vi "HHSetInpChan.vi"(0 "Channel":i32=1 min=1 max=8 step=1, 1 "CFD Level":i32=50 min=-1300 max=400 step=10, 2 "CFD ZeroX":i32=10 min=-1300 max=400 step=10, 3 "Offset":i32=10 min=-1300 max=400 step=10, 4 "DeviceIndex":i32) -> (5 "Error":bool)   [LabVIEW 2009]
uses:
  hhlib.dll
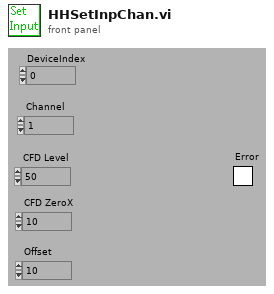
[diagram p1: front panel]
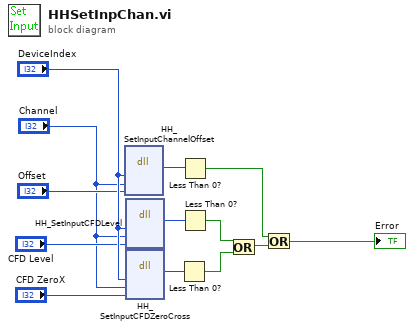
[diagram p0: block diagram]
diagram:
  n1 = dll-call lib="C:/Programme/Anwendungen/DAQLinescan_HH/hhlib.dll" fn="HH_SetInputChannelOffset"("devidx"="DeviceIndex", "channel"="Channel", "offset"="Offset") -> (w11:i32)  [unwired: 6 in, 2 out]
  n2 = dll-call lib="C:/Programme/Anwendungen/DAQLinescan_HH/hhlib.dll" fn="HH_SetInputCFDLevel"("devidx"="DeviceIndex", "channel"="Channel", "level"="CFD Level") -> (w10:i32)  [unwired: 6 in, 2 out]
  n3 = dll-call lib="C:/Programme/Anwendungen/DAQLinescan_HH/hhlib.dll" fn="HH_SetInputCFDZeroCross"("devidx"="DeviceIndex", "channel"="Channel", "Level"="CFD ZeroX") -> (w9:i32)  [unwired: 6 in, 2 out]
  n4 = Less Than 0?(x=w9) -> (x < 0?=w8:bool)
  n5 = Less Than 0?(x=w11) -> (x < 0?=w6:bool)
  n6 = Less Than 0?(x=w10) -> (x < 0?=w13:bool)
  n7 = Or(x=w13, y=w8) -> (x .or. y?=w12:bool)
  n8 = Or(x=w6, y=w12) -> (x .or. y?=→"Error":bool)
